vi "TxRx.vi"(5 "Timeout (Ms)":u32, 6 "Receive?":bool=TRUE, 7 "Wait Before Read (Ms)":u32, 8 "error in":errorcluster, 10 "Tx Message":string, 11 "VISA Resource Name In":refnum<visa-resource-name>) -> (0 "error out":errorcluster, 2 "Rx Message":string, 3 "VISA Resource Name Out":refnum<visa-resource-name>)   [LabVIEW 2020, in "MicroPython.lvlib"]
doc: "This VI will transmit a message over the serial port and optionally wait for a response from the target device.\nIf waiting for a reponse, we will listen as long as the device is sending data or until with have received more than some maximum threshold (set in the block diagram. See MaxRxLength).\nAfter each bundle of data is received, we will wait for a period equal to \"Wait Before Read (Ms)\" before trying to read more.\nIf we have waited for \"Wait Before Read (Ms)\" and we notice timeout is reached or we have at least one byte received, we will assume the device is done sending messages, and we will leave."
uses:
  MicroPython.lvlib
panel:
  out "Rx Length":i32
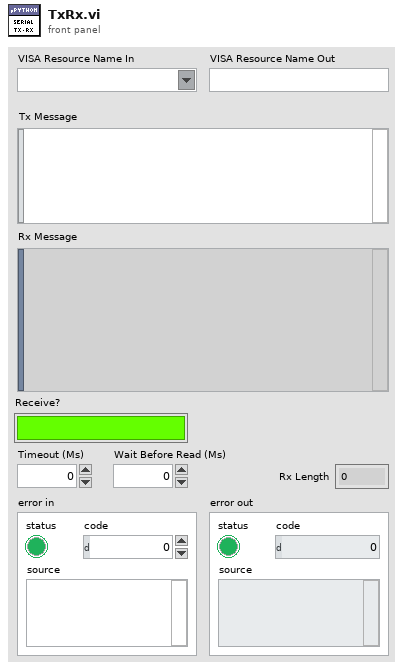
[diagram p1: front panel]
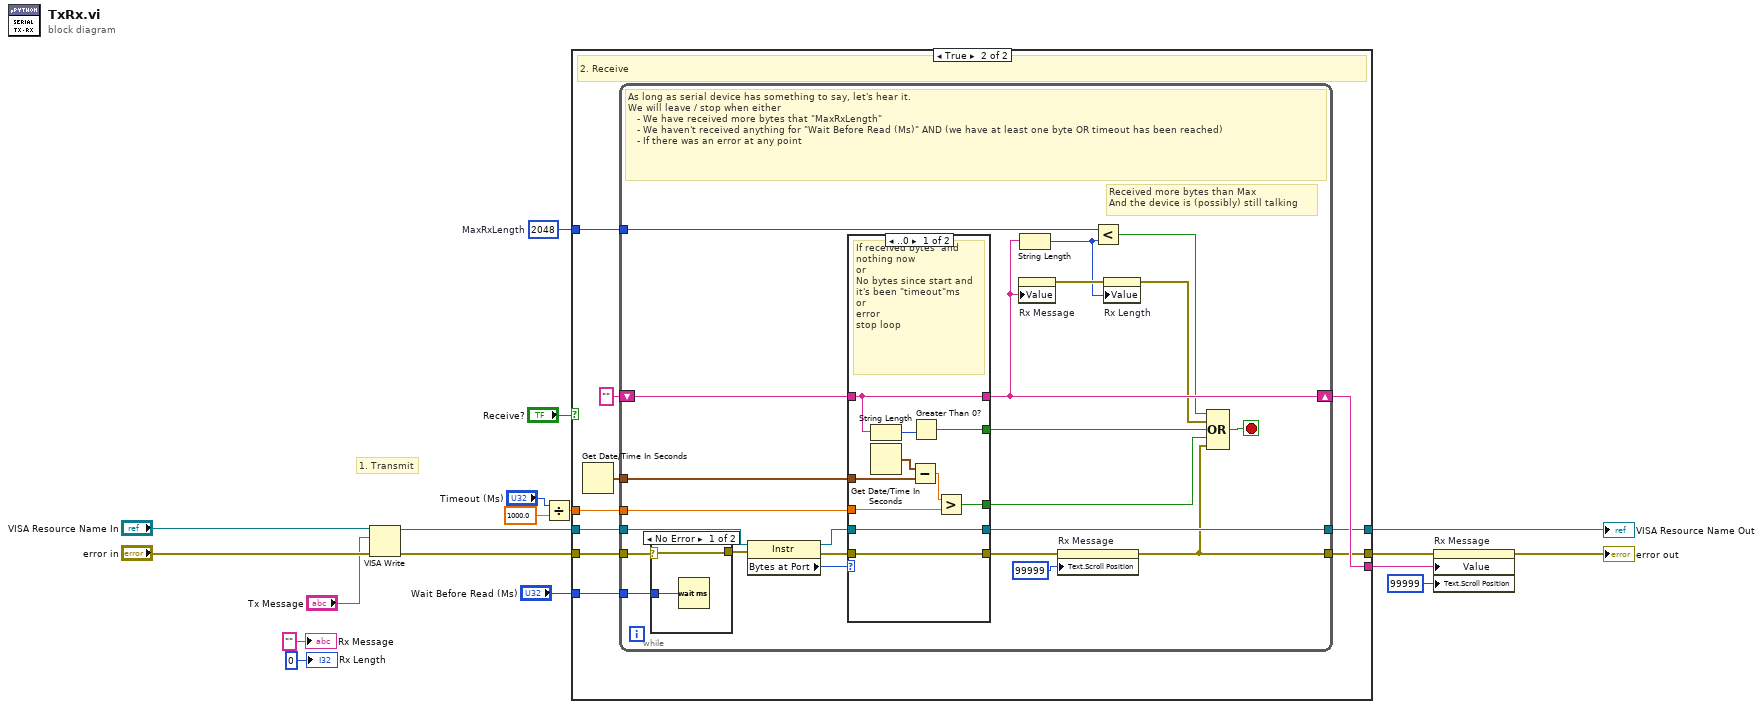
[diagram p0: block diagram]
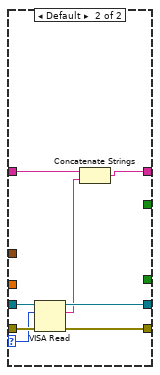
[diagram p4: hidden frame]
diagram:
  w6 = 2048  # MaxRxLength
  # "1. Transmit"
  n1 = VISA Write(VISA resource name="VISA Resource Name In", write buffer="Tx Message", error in (no error)="error in") -> (VISA resource name out=w15:refnum<visa-resource-name>, error out=w14:errorcluster)  [unwired: 1 out]
  n2 = Divide(x="Timeout (Ms)", y=1000.0) -> (x/y=w1:dbl)
  n3 = case shown="True" "Receive?" {
    tunnel: w15 -> [w20 w30]
    tunnel: w14 -> [w19 w28]
    tunnel: "Wait Before Read (Ms)" -> [_ w27]
    tunnel: [_ w25] -> w12
    tunnel: [w19 w24] -> w10
    tunnel: [w20 w23] -> w9
    tunnel: w6 -> [_ w22]
    tunnel: w1 -> [_ w21]
    frame False {
      # "Do not wait for reply from target device"
    }
    frame True {
      # "2. Receive"
      n4 = Get Date/Time In Seconds() -> (seconds since 1Jan1904=w26:timestamp)
      n5 = while {
        tunnel: [w36] -> w24
        tunnel: w30 -> [w53]
        shift-right: [w39] -> w25
        shift-left: "" -> [w45]
        tunnel: [w51] -> w23
        tunnel: w28 -> [w48]
        tunnel: w27 -> [w47]
        tunnel: w26 -> [w44]
        tunnel: w22 -> [w33]
        tunnel: w21 -> [w31]
        stop <- w41 stop-if-true
        # "Received more bytes than Max\nAnd the device is (possibly) still talking"
        # "As long as serial device has something to say, let's hear it.\nWe will leave / stop when either \n   - We have received more bytes that \"MaxRxLength\"\n   - We haven't received anything for \"Wait Before Read (Ms)\" AND (we have at least one byte OR timeout has been reached) \n   - If there was an error at any point"
        n6 = case shown="No Error" w48 {
          selector: w48 -> [w54 w56]
          tunnel: w47 -> [w55 _]
          tunnel: [w54 w56] -> w46
          frame No Error {
            n7 = Wait (ms)(milliseconds to wait=w55) -> ()  [unwired: 1 out]
          }
          frame Error {
          }
        }
        n8 = property on="Property Node" class="Instr"(reference=w53, error in=w46) -> (reference out=w52:refnum<visa-resource-name>, error out=w50:errorcluster, "Bytes at Port"=w49:u32)
        n9 = case shown="..0" w49 {
          selector: w49 -> [_ w70]
          tunnel: w52 -> [w66 w74]
          tunnel: [w66 w73] -> w51
          tunnel: w50 -> [w65 w72]
          tunnel: [w65 w71] -> w37
          tunnel: [w64 w69] -> w39
          tunnel: w45 -> [w64 w68]
          tunnel: w44 -> [w61 _]
          tunnel: w31 -> [w59 _]
          tunnel: [w58 _] -> w43
          tunnel: [w57 _] -> w42
          frame ..0 {
            # "If received bytes  and nothing now\nor\nNo bytes since start and it's been \"timeout\"ms\nor \nerror\nstop loop"
            n10 = String Length(string=w64) -> (length=w63:i32)
            n11 = Get Date/Time In Seconds() -> (seconds since 1Jan1904=w62:timestamp)
            n12 = Subtract(x=w62, y=w61) -> (x-y=w60:dbl)
            n13 = Greater Than 0?(x=w63) -> (x > 0?=w58:bool)
            n14 = Greater?(x=w60, y=w59) -> (0:w57:bool)
          }
          frame Default {
            n15 = VISA Read(VISA resource name=w74, byte count=w70, error in (no error)=w72) -> (VISA resource name out=w73:refnum<visa-resource-name>, read buffer=w67:string, error out=w71:errorcluster)  [unwired: 1 out]
            n16 = Concatenate Strings(w68, w67) -> (w69:string)
          }
        }
        n17 = property on="Rx Message" class="Str"("Value"=w39) -> (error out=w38:errorcluster)  [unwired: 2 in, 1 out]
        n18 = String Length(string=w39) -> (length=w32:i32)
        n19 = property on="Rx Message" class="Str"(error in=w37, "Text.Scroll Position"=u32 99999 ("byte count")) -> (error out=w36:errorcluster)  [unwired: 1 in, 1 out]
        n20 = Less?(x=w33, y=w32) -> (x < y?=w34:bool)
        n21 = property on="Rx Length" class="DigNum (strict)"(error in=w38, "Value"=w32) -> (error out=w35:errorcluster)  [unwired: 1 in, 1 out]
        n22 = Compound Arithmetic op=OR(w34, w35, w43, w42, w36) -> (w41:bool)
      }
    }
  }
  "VISA Resource Name Out" <- w9
  n23 = property on="Rx Message" class="Str"(error in=w10, "Value"=w12, "Text.Scroll Position"=u32 99999 ("byte count")) -> (error out=→"error out":errorcluster)  [unwired: 1 in, 1 out]
  "Rx Length" <- 0 ("Rx Length")
  "Rx Message" <- "" ("Rx Message")
